vi "Set Rmb.vi"(8 "error in (no error)":errorcluster, 10 "enable rmb user":bool, 11 "[Data] Recent User in":refnum<class "[User] Recent Login.lvclass">) -> (0 "error out":errorcluster, 3 "[Data] Recent User out":refnum<class "[User] Recent Login.lvclass">)   [LabVIEW 2020, in "[User] Recent Login.lvclass"]
uses:
  [User] Recent Login.lvclass
  [User] Recent Login.lvclass/[User] Recent Login.ctl
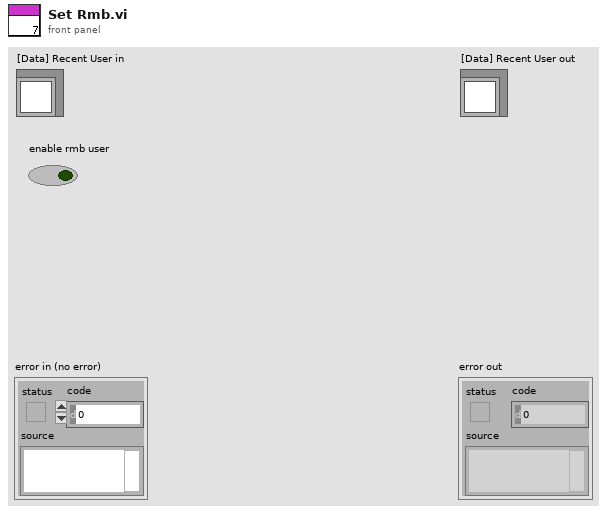
[diagram p1: front panel]
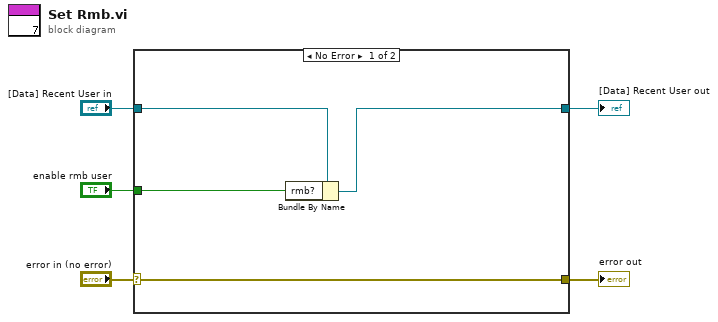
[diagram p0: block diagram]
diagram:
  n1 = case shown="No Error" "error in (no error)" {
    selector: "error in (no error)" -> [w9 w11]
    tunnel: [w9 w11] -> w4
    tunnel: [w6 w10] -> w2
    tunnel: "[Data] Recent User in" -> [w8 w10]
    tunnel: "enable rmb user" -> [w7 _]
    frame No Error {
      n2 = Bundle By Name(cluster=w8, "rmb?"=w7) -> (w6:refnum<class "[User] Recent Login.lvclass">)
    }
    frame Error {
    }
  }
  "error out" <- w4
  "[Data] Recent User out" <- w2
